vi "generate 1 cycle.vi"(8 "error in (no error)":errorcluster caption="에러 입력(에러 없음)", 11 "Square Wave 입력":refnum<class "Square Wave.lvclass">) -> (0 "error out":errorcluster caption="에러 출력", 2 "waveform":waveform(dbl), 3 "Square Wave 출력":refnum<class "Square Wave.lvclass">)   [LabVIEW 2020, in "Square Wave.lvclass"]
uses:
  Square Wave.lvclass
  Waveform Gen/Waveform Gen.lvclass/Waveform Gen.ctl
  Waveform Obj/Waveform Obj.lvclass/Waveform Obj.ctl
  Square Wave.lvclass/Square Wave.ctl
  Waveform Gen/Accessors/Read scale.vi
  Waveform Obj/Accessors/Read sampling rate.vi
  Waveform Gen/Accessors/Read frequency.vi
  Accessors/Read slope length.vi
  Accessors/Read slope type.vi
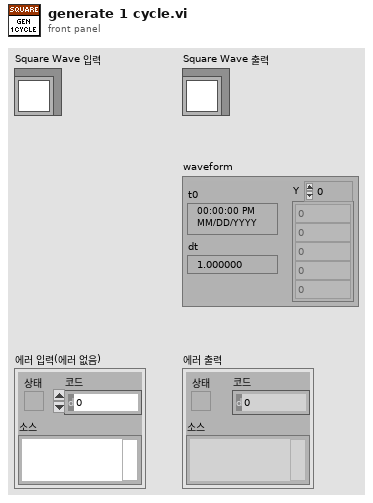
[diagram p1: front panel]
types:
  T1 = typedef "Square Wave.lvclass/Slope Type.ctl" = enum16{"None", "Lin.", "Exp."}
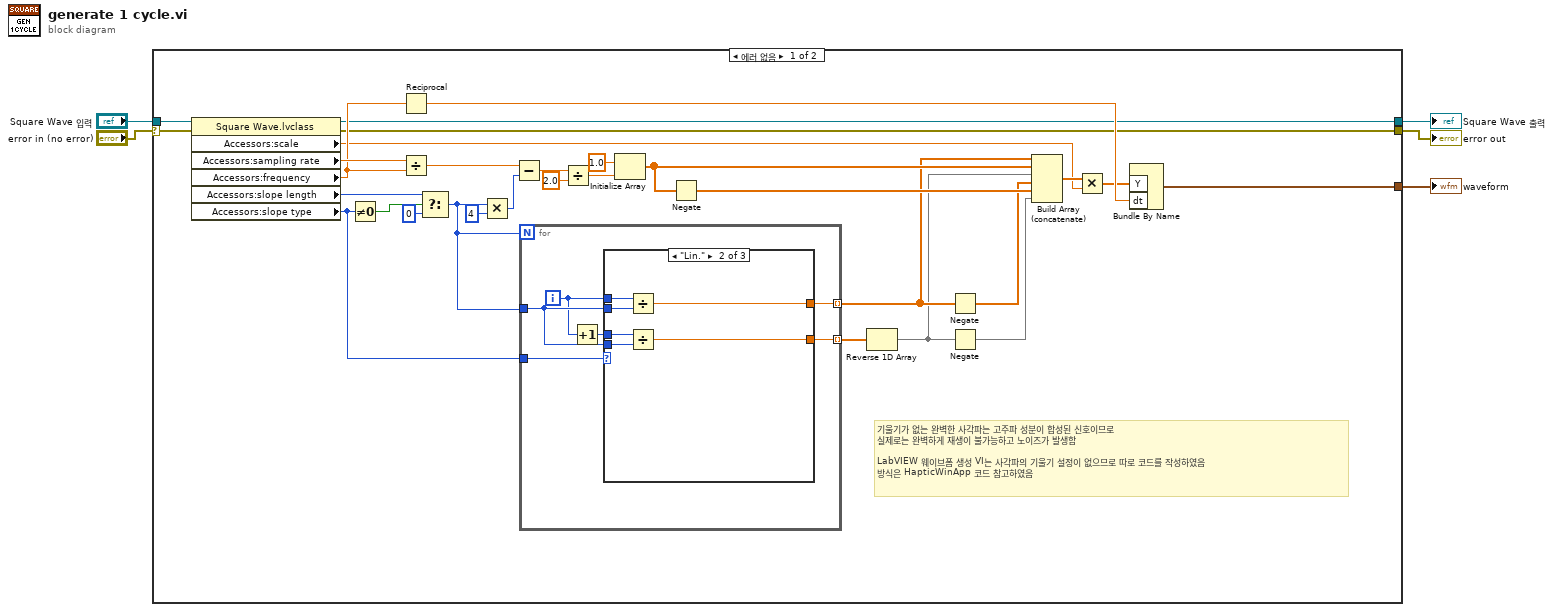
[diagram p0: block diagram]
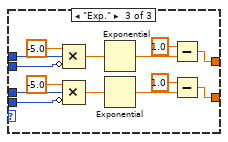
[diagram p3: hidden frame]
diagram:
  n1 = case shown="에러 없음" "error in (no error)" {
    selector: "error in (no error)" -> [w19 w62]
    tunnel: [w7 w62] -> w4
    tunnel: [w8 w63] -> w3
    tunnel: "Square Wave 입력" -> [w22 w63]
    tunnel: [w6 _] -> w1
    frame No Error {
      # "기울기가 없는 완벽한 사각파는 고주파 성분이 합성된 신호이므로 \n실제로는 완벽하게 재생이 불가능하고 노이즈가 발생함\n\nLabVIEW 웨이브폼 생성 VI는 사각파의 기울기 설정이 없으므로 따로 코드를 작성하였음\n방식은 HapticWinApp 코드 참고하였음"
      n2 = property class="Square Wave.lvclass"(reference=w22, error in=w19) -> (reference out=w8:refnum<class "Square Wave.lvclass">, error out=w7:errorcluster, "Accessors:scale"=w9:dbl, "Accessors:sampling rate"=w21:dbl, "Accessors:frequency"=w17:dbl, "Accessors:slope length"=w20:u32, "Accessors:slope type"=w14:T1)
      n3 = Not Equal To 0?(x=w14) -> (x != 0?=w13:bool)
      n4 = Reciprocal(x=w17) -> (1/x=w16:dbl)
      n5 = Divide(x=w21, y=w17) -> (x/y=w35:dbl)
      n6 = Select(t=w20, s=w13, f=u32 0) -> (s? t:f=w15:u32)
      n7 = Multiply(x=w15, y=u32 4 ("x")) -> (x*y=w33:u32)
      n8 = Subtract(x=w35, y=w33) -> (x-y=w32:dbl)
      n9 = for {
        N: w15 -> [_]
        tunnel: w15 -> [w40]
        tunnel: [w41] -> w27 mode=indexing
        tunnel: [w37] -> w24 mode=indexing
        tunnel: w14 -> [w36]
        i -> [w39]
        n10 = Increment(x=w39) -> (x+1=w38:i32)
        n11 = case shown="\"Lin.\"" w36 {
          tunnel: w39 -> [_ w47 w59]
          tunnel: w40 -> [_ w46 w58]
          tunnel: [_ w45 w55] -> w41
          tunnel: w40 -> [_ w43 w50]
          tunnel: w38 -> [_ w44 w49]
          tunnel: [_ w42 w48] -> w37
          frame "None", Default {
          }
          frame "Lin." {
            n12 = Divide(x=w47, y=w46) -> (x/y=w45:dbl)
            n13 = Divide(x=w44, y=w43) -> (x/y=w42:dbl)
          }
          frame "Exp." {
            n14 = Compound Arithmetic op=MULTIPLY(-5.0 ("x"), w59, invert w58) -> (w57:dbl)
            n15 = Compound Arithmetic op=MULTIPLY(-5.0 ("x"), w49, invert w50) -> (w53:dbl)
            n16 = Exponential(1:w57) -> (0:w56:dbl)
            n17 = Exponential(1:w53) -> (0:w54:dbl)
            n18 = Subtract(x=1.0, y=w56) -> (x-y=w55:dbl)
            n19 = Subtract(x=1.0, y=w54) -> (x-y=w48:dbl)
          }
        }
      }
      n20 = Divide(x=w32, y=2.0) -> (x/y=w30:dbl)
      n21 = Initialize Array(1.0 ("원소"), w30) -> (w29:dbl[])
      n22 = Negate(x=w29) -> (-x=w28:dbl[])
      n23 = Reverse 1D Array(array=w24) -> (reversed array=w23:dbl[])
      n24 = Negate(x=w27) -> (-x=w26:dbl[])
      n25 = Negate(x=w23) -> (-x=w25:dbl[])
      n26 = Build Array (concatenate)(w27, w29, w23, w26, w28, w25) -> (w18:dbl[])
      n27 = Multiply(x=w18, y=w9) -> (x*y=w10:dbl[])
      n28 = Bundle By Name("Y"=w10, "dt"=w16) -> (w6:waveform(dbl))  [unwired: 1 in]
    }
    frame Error {
    }
  }
  "error out" <- w4
  "Square Wave 출력" <- w3
  "waveform" <- w1
